vi "Read target.vi"(8 "error in (no error)":errorcluster, 11 "WaveFrontTargetPosition in":refnum<class "WaveFrontTargetPosition.lvclass">) -> (0 "error out":errorcluster, 2 "TCSGuiderStatus.lvlib:GWTargetPositionParameters.lvclass":refnum<class "GWTargetPositionParameters.lvclass">, 3 "WaveFrontTargetPosition out":refnum<class "WaveFrontTargetPosition.lvclass">)   [LabVIEW 2014, in "TCSDataDefinitions.lvlib" / "TCSWFSStatus.lvlib" / "WaveFrontTargetPosition.lvclass"]
uses:
  WaveFrontTargetPosition.lvclass
  TCSGuiderStatus/GWTargetPositionParameters/GWTargetPositionParameters.lvclass
  WaveFrontTargetPosition.lvclass/WaveFrontTargetPosition.ctl
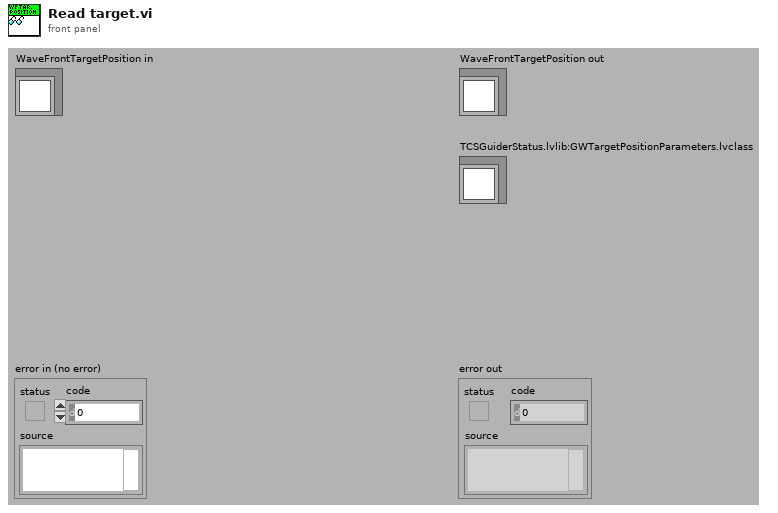
[diagram p1: front panel]
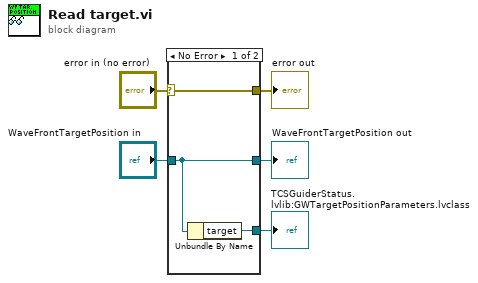
[diagram p0: block diagram]
diagram:
  n1 = case shown="No Error" "error in (no error)" {
    selector: "error in (no error)" -> [w8 w9]
    tunnel: [w8 w9] -> w4
    tunnel: [w7 w10] -> w2
    tunnel: "WaveFrontTargetPosition in" -> [w7 w10]
    tunnel: [w6 _] -> w1
    frame No Error {
      n2 = Unbundle By Name(w7) -> ("target"=w6:refnum<class "GWTargetPositionParameters.lvclass">)
    }
    frame Error {
    }
  }
  "error out" <- w4
  "WaveFrontTargetPosition out" <- w2
  "TCSGuiderStatus.lvlib:GWTargetPositionParameters.lvclass" <- w1
